vi "Create Test Radio.vi"(8 "error in (no error)":errorcluster, 11 "LCM Single-Up MTS Test in":refnum<class "LCM Single-Up MTS Test.lvclass">) -> (0 "error out":errorcluster, 3 "Test Radio":refnum<class "SC Manufacturing Test.lvclass">)   [LabVIEW 2015, in "LCM Single-Up MTS Test.lvclass"]
uses:
  LCM Single-Up MTS Test.lvclass
  Classes/Manufacturing Test/Class/SC Manufacturing Test.lvclass
  Classes/Test Recipe/Class/Test Recipe.lvclass
  <vilib>/Cree, Inc/Cree Test Framework/Classes/Base Objects/Base Class/Base Class/Base Class.lvclass
  Classes/Application/Class/Application.lvclass
  Test Class/Test Class.lvclass
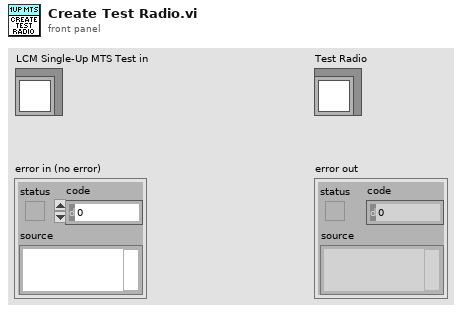
[diagram p1: front panel]
types:
  T1 = typedef "Application.lvlib/App Properties.lvclass/Class Properties -- Cluster.ctl" = cluster{"UUT Info":T2[], "Test Information":refnum<vi>, "Test Complete Event":refnum<user-event>, "Shop Floor System":refnum<class "Shop Floor System.lvclass">, "Gold Board":refnum<class "Golden Board.lvclass">, "Test Recipe":refnum<class "Test Recipe.lvclass">, "Instruments":refnum<class "Instrument.lvclass">[], "Mode":T3, "Test Results":cluster{"Pass":bool[], "Fail Codes":string[]}, "Station Config":refnum<class "Station Config.lvclass">}
  T2 = typedef "Application.lvlib/App Properties.lvclass/UUT Reference -- Cluster.ctl" = cluster{"Serial Number Reference":refnum<vi>, "Status Message Reference":refnum<vi>}
  T3 = typedef "Application.lvlib/Application.lvclass/Op Mode -- Enum.ctl" = u16
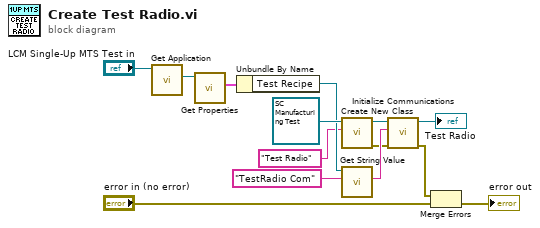
[diagram p0: block diagram]
diagram:
  n1 = call "Get Application.vi"("Test Class in"="LCM Single-Up MTS Test in") -> ("Application.lvlib:Application.lvclass"=w8:refnum<class "Application.lvclass">)  [unwired: 9 in, 1 out]
  n2 = call "Get Properties.vi"("Acrobat Template in"=w8) -> ("Class Properties"=w9:T1)  [unwired: 8 in, 2 out]
  n3 = Unbundle By Name(w9) -> ("Test Recipe"=w7:refnum<class "Test Recipe.lvclass">)
  n4 = call <vilib>:"Create New Class.vi"("Name"="Test Radio", "Base Class in"=refnum<class "SC Manufacturing Test.lvclass"> refnum ("SC Manufacturing Test.lvlib:SC Manufacturing Test.lvclass")) -> ("error out"=w11:errorcluster, "Base Class out"=w12:refnum<class "SC Manufacturing Test.lvclass">)  [unwired: 8 in]
  n5 = call "Get String Value.vi"("Name"="TestRadio Com", "Test Recipe in"=w7) -> ("Value"=w13:string)  [unwired: 7 in, 2 out]
  n6 = call "Initialize Communications.vi"("error in (no error)"=w11, "COM Port"=w13, "Acrobat Template in"=w12) -> ("error out"=w1:errorcluster, "Acrobat Template out"=→"Test Radio":refnum<class "SC Manufacturing Test.lvclass">)  [unwired: 7 in]
  n7 = Merge Errors(w1, "error in (no error)") -> (→"error out":errorcluster)
